vi "Get Time Door Has Been Open.vi"(8 "error in (no error)":errorcluster, 11 "Timed Door in":refnum<class "Timed Door.lvclass">) -> (0 "error out":errorcluster, 2 "Elapsed Time (seconds)":dbl, 3 "Timed Door out":refnum<class "Timed Door.lvclass">)   [LabVIEW 2018, in "Timed Door.lvclass"]
uses:
  Timed Door.lvclass
  Timed Door.lvclass/Timed Door.ctl
  Timer/Timer.lvclass
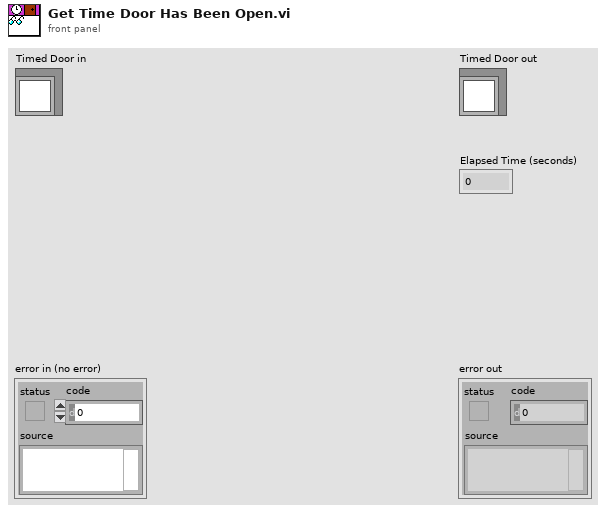
[diagram p1: front panel]
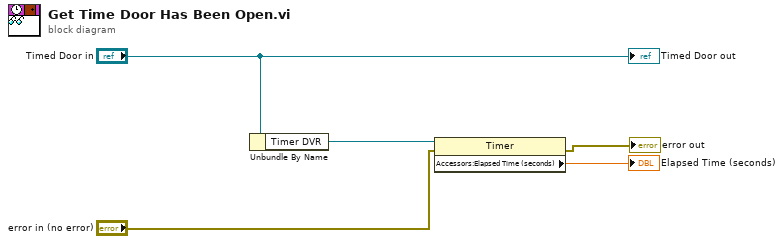
[diagram p0: block diagram]
diagram:
  n1 = Unbundle By Name("Timed Door in") -> ("Timer DVR"=w4:refnum<data-value>)
  n2 = property class="Timer"(reference=w4, error in="error in (no error)") -> (error out=→"error out":errorcluster, "Accessors:Elapsed Time (seconds)"=→"Elapsed Time (seconds)":dbl)  [unwired: 1 out]
  "Timed Door out" <- "Timed Door in"
